vi "filtersignalbak.vi"(0 "Array":dbl[](array[numeric]), 1 "m":dbl, 2 "3s":dbl) -> (6 "Waveform Chart 2":dbl[](graph), 7 "Numeric":i32)   [LabVIEW 2014]
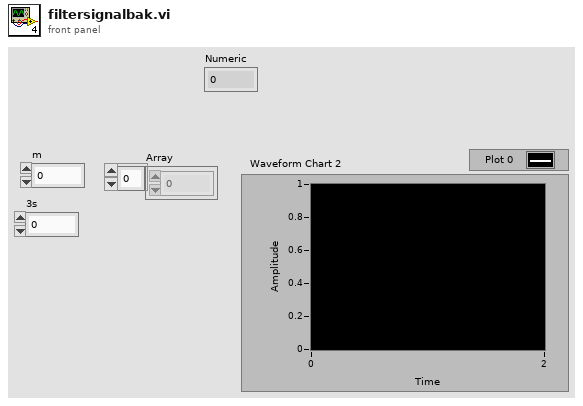
[diagram p1: front panel]
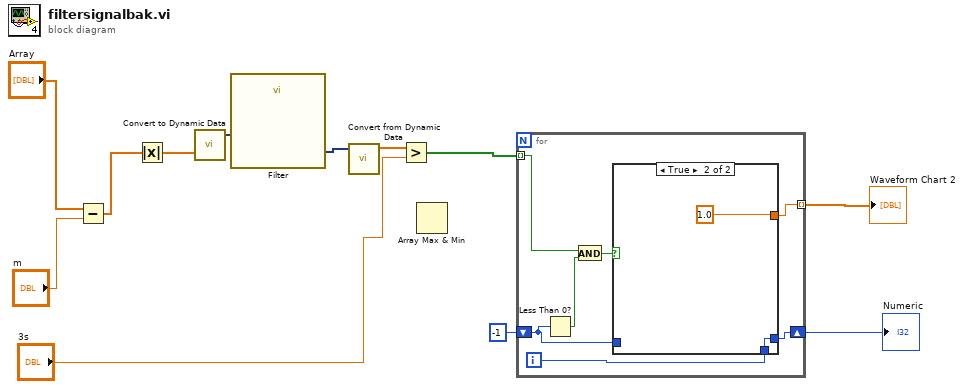
[diagram p0: block diagram]
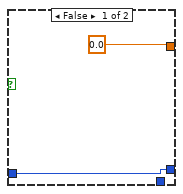
[diagram p2: hidden frame]
diagram:
  n1 = Subtract(x="Array", y="m") -> (x-y=w12:dbl[])
  n2 = Absolute Value(x=w12) -> (abs(x)=w10:dbl[])
  n3 = call "Convert to Dynamic Data"("Array"=w10) -> ("Dynamic Data Type"=w8:dynamicdata)  [unwired: 3 in]
  n4 = call "Filter"("Signal"=w8) -> ("Filtered Signal"=w7:dynamicdata)  [unwired: 9 in, 1 out]
  n5 = call "Convert from Dynamic Data"("Dynamic Data Type"=w7) -> ("Array"=w5:dbl[])  [unwired: 3 in]
  n6 = Greater?(x=w5, y="3s") -> (0:w3:bool[])
  n7 = Array Max & Min() -> ()  [unwired: 1 in, 4 out]
  n8 = for {
    shift-right: [w16] -> w2
    shift-left: -1 -> [w15]
    tunnel: w3 -> [w18] mode=indexing
    tunnel: [w13] -> w1 mode=indexing
    i -> [w14]
    n9 = Less Than 0?(x=w15) -> (x < 0?=w17:bool)
    n10 = And(x=w18, y=w17) -> (x .and. y?=w19:bool)
    n11 = case shown="True" w19 {
      tunnel: [w21 w23] -> w16
      tunnel: w15 -> [w21 _]
      tunnel: w14 -> [_ w23]
      tunnel: [0.0 ("f") 1.0 ("t")] -> w13
      frame False {
      }
      frame True {
      }
    }
  }
  "Numeric" <- w2
  "Waveform Chart 2" <- w1
